vi "CloseConnection.vi"(8 "error in (no error)":errorcluster, 11 "Modbus In":refnum<class "Modbus.lvclass">) -> (0 "error out":errorcluster, 3 "Modbus Out":refnum<class "Modbus.lvclass">)   [LabVIEW 2019, in "Modbus.lvclass"]
uses:
  Modbus.lvclass
  Modbus.lvclass/Modbus.ctl
  <vilib>/NI/Modbus Library/API/Master/Modbus Master.lvclass
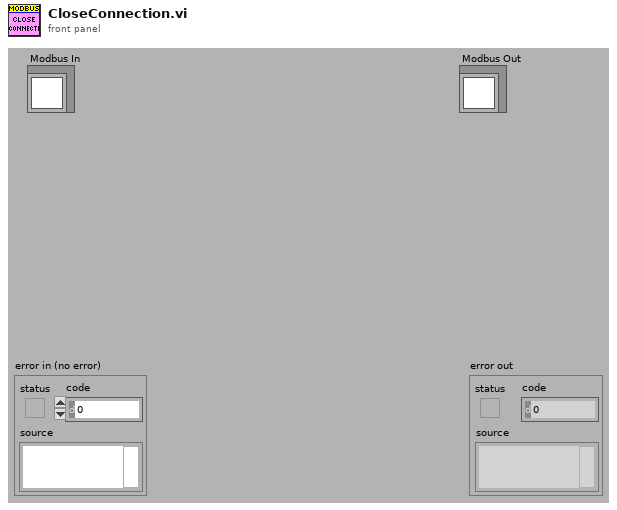
[diagram p1: front panel]
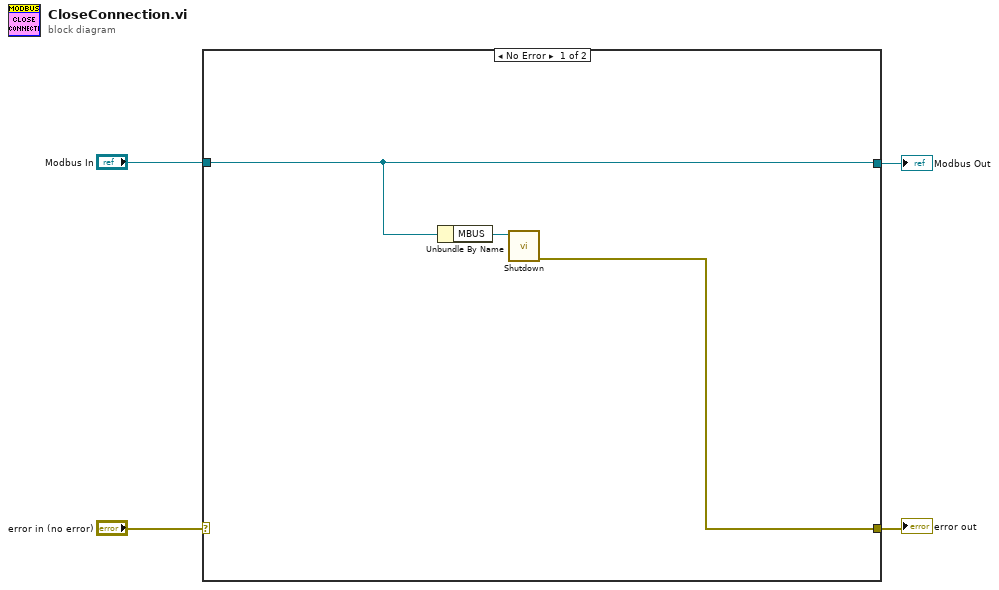
[diagram p0: block diagram]
diagram:
  n1 = case shown="No Error" "error in (no error)" {
    selector: "error in (no error)" -> [_ w9]
    tunnel: [w5 w9] -> w3
    tunnel: [w7 w8] -> w1
    tunnel: "Modbus In" -> [w7 w8]
    frame No Error {
      n2 = Unbundle By Name(w7) -> ("MBUS"=w6:refnum<class "Modbus Master.lvclass">)
      n3 = call-dynamic "Shutdown.vi"("Modbus master in"=w6) -> ("error out"=w5:errorcluster)  [unwired: 10 in]
    }
    frame Error {
    }
  }
  "error out" <- w3
  "Modbus Out" <- w1
